vi "禹山电导率_获取温度和测量值.vi"(8 "error in (no error)":errorcluster caption="错误输入（无错误）", 11 "MB session in":refnum<class "MB_Master.lvclass">) -> (0 "error out":errorcluster caption="错误输出", 2 "输出值":cluster{"温度测量值":sgl, "电导率":sgl, "错误标志":u16} {"错误标志" items=["NO Error"=0, "量程切换错误标识"=255]}, 3 "MB session out":refnum<class "MB_Master.lvclass">)   [LabVIEW 2016, in "斯坦道多参数.lvlib"]
uses:
  <vilib>/Plasmionique/MB Master/MB_Master/MB_Master.lvclass
  <vilib>/Plasmionique/MB Master/MB Master.lvlib
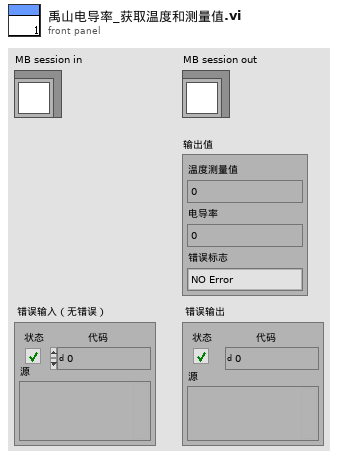
[diagram p1: front panel]
types:
  T1 = cluster{"pH":u32, "DO":u32, "Cond":u32, "Turb":u32, "叶绿素a":u32, "藻密度":u32, "ORP":u32, "COD":u32, "氯化物":u32, "氨氮":u32, "水中油":u32, "悬浮物":u32, "余氯":u32}
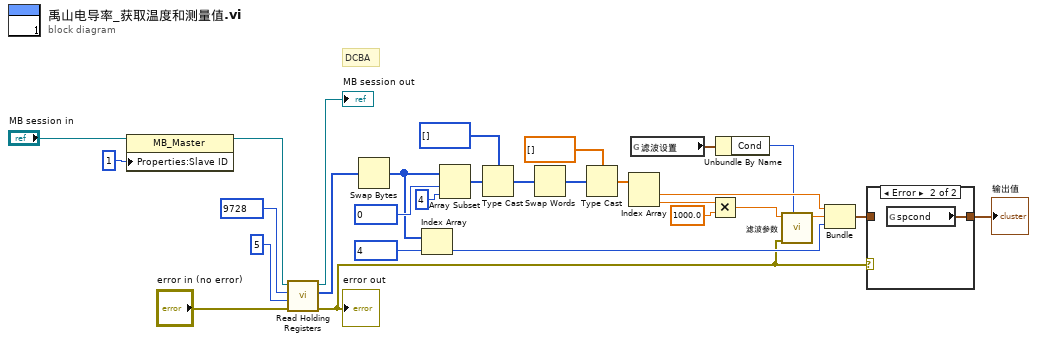
[diagram p0: block diagram]
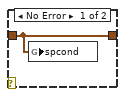
[diagram p2: hidden frame]
diagram:
  # "DCBA"
  n1 = property class="MB_Master"(reference="MB session in", "Properties:Slave ID"=u16 1 ("y")) -> (reference out=w21:refnum<class "MB_Master.lvclass">)  [unwired: 1 in, 1 out]
  n2 = call <vilib>:"Read Holding Registers.vi"("error in (no error)"="error in (no error)", "quantity"=u16 5, "starting address"=u16 9728, "MB session in"=w21) -> ("error out"=w1:errorcluster, "Registers"=w19:u16[], "MB session out"=→"MB session out":refnum<class "MB_Master.lvclass">)  [unwired: 5 in]
  "error out" <- w1
  n3 = Swap Bytes(anything=w19) -> (byte swapped=w10:u16[])
  n4 = Index Array(array=w10, index=u16 4 ("starting address")) -> (element=w9:u16)
  n5 = Array Subset(array=w10, index=u16 0 ("starting address"), length=4 ("长度")) -> (w14:u16[])
  n6 = Type Cast(type=u32[] [] ("数组 2"), x=w14) -> (*(type *) &x=w25:u32[])
  n7 = Swap Words(1:w25) -> (0:w27:u32[])
  n8 = Type Cast(type=sgl[] [] ("数组 2"), x=w27) -> (*(type *) &x=w23:sgl[])
  n9 = Index Array(array=w23) -> (element #1=w18:sgl, element #2=w17:sgl)  [unwired: 2 in]
  n10 = global read "断电保存变量.vi" "滤波设置"() -> (w4:T1)
  n11 = Multiply(x=w17, y=sgl 1000.0) -> (x*y=w6:sgl)
  n12 = Unbundle By Name(w4) -> ("Cond"=w3:u32)
  n13 = call "滤波参数.vi"("滤波次数"=w3, "error in (no error)"=w1, "x"=w6) -> ("mode"=w5:dbl)  [unwired: 7 in, 1 out]
  n14 = Bundle("数值"=w18, "mode"=w5, w9) -> (w15:cluster{"数值":sgl, "mode":dbl, u16})  [unwired: 1 in]
  n15 = case shown="Error" w1 {
    tunnel: w15 -> [w30 _]
    tunnel: [w30 w31] -> w2
    frame No Error {
      n16 = global write "禹山过程全局变量.vi" "spcond"(w30) -> ()
    }
    frame Error {
      n17 = global read "禹山过程全局变量.vi" "spcond"() -> (w31:cluster{"温度测量值":sgl, "测量值":sgl, "错误标志":u16})
    }
  }
  "输出值" <- w2
